vi "Thingworx_Example2.vi"() -> ()   [LabVIEW 2016]
panel:
  in  "stop":bool
  out "Property":T1
  out "Table Control":string[][](table)=[["test", "test", "STRING"]]
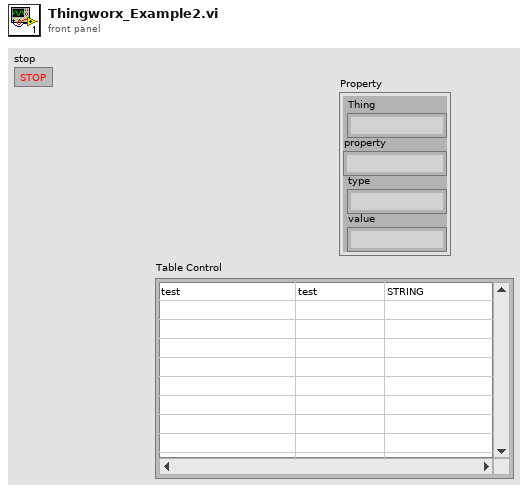
[diagram p1: front panel]
types:
  T1 = cluster{"Thing":string, "property":string, "type":string, "value":string}
  T2 = cluster{"Thing":string, "property":string, "type":string, string}
  T3 = typedef "Device.ctl" = cluster{"Name":string, "BaseURL":string, "AppKey":string, "Headers":string[], "Timeout":i32, "Identifier":string, "Password":string, "Comments":string, "Handle":u32, "# Handles":i32}
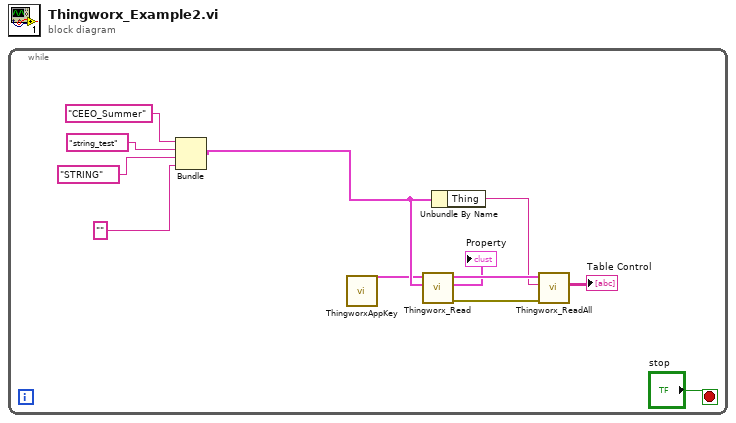
[diagram p0: block diagram]
diagram:
  n1 = while {
    stop <- "stop" stop-if-true
    n2 = Bundle("Thing"="CEEO_Summer", "property"="string_test", "type"="STRING", "") -> (w4:T2)  [unwired: 1 in]
    n3 = call "ThingworxAppKey.vi"() -> ("Device Out"=w3:T3)  [unwired: 11 in]
    n4 = call "Thingworx_Read.vi"("Property In"=w4, "Device in"=w3) -> ("error out"=w11:errorcluster, "Property"=→"Property":T1, "Device Out"=w12:T3)  [unwired: 7 in]
    n5 = Unbundle By Name(w4) -> ("Thing"=w8:string)
    n6 = call "Thingworx_ReadAll.vi"("error in (no error)"=w11, "Thing"=w8, "Device in"=w12) -> ("Properties"=→"Table Control":string[][])  [unwired: 6 in, 2 out]
  }
